vi "specu1a 1.0.0 String to 16xU8 Cluster.vi"(7 "String in":string, 9 "offset (0)":i32) -> (8 "16xU8 Cluster":T1)   [LabVIEW 2010]
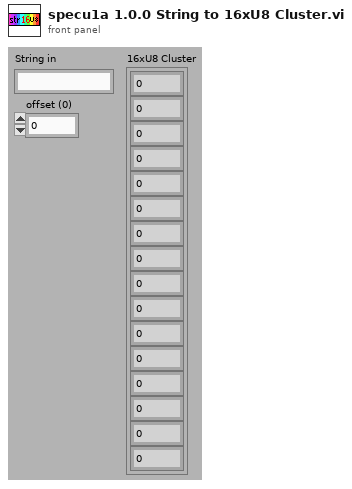
[diagram p1: front panel]
types:
  T1 = cluster{u8, u8, u8, u8, u8, u8, u8, u8, u8, u8, u8, u8, u8, u8, u8, u8}
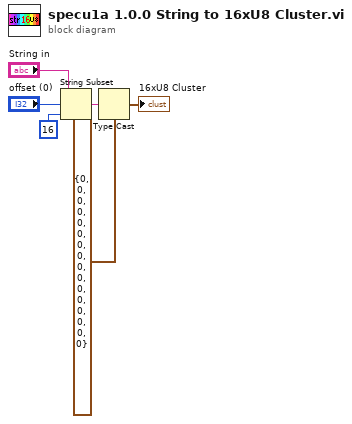
[diagram p0: block diagram]
diagram:
  n1 = String Subset(string="String in", offset (0)="offset (0)", length (rest)=16) -> (substring=w1:string)
  n2 = Type Cast(type=T1 {0, 0, 0, 0, 0, 0, 0, 0, 0, 0, 0, 0, 0, 0, 0, 0}, x=w1) -> (*(type *) &x=→"16xU8 Cluster":T1)
